vi "Joystick xor switch.vi"(10 "Down":bool, 11 "Up":bool) -> (3 "Output":i32)   [LabVIEW 2014]
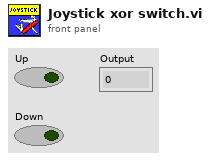
[diagram p1: front panel]
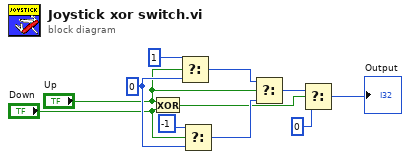
[diagram p0: block diagram]
diagram:
  w9 = 0
  n1 = Exclusive Or(1:"Down", 2:"Up") -> (0:w3:bool)
  n2 = Select(t=1, s="Up", f=w9) -> (s? t:f=w11:i32)
  n3 = Select(t=-1, s="Down", f=w9) -> (s? t:f=w10:i32)
  n4 = Select(t=w11, s="Up", f=w10) -> (s? t:f=w5:i32)
  n5 = Select(t=w5, s=w3, f=0) -> (s? t:f=→"Output":i32)
